vi "error_messages.vi"(8 "error in (no error)":errorcluster) -> ()   [LabVIEW 2015]
uses:
  <vilib>/Utility/error.llb/DialogType.ctl
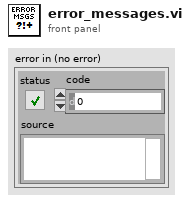
[diagram p1: front panel]
types:
  T1 = typedef "DialogType.ctl" = u16
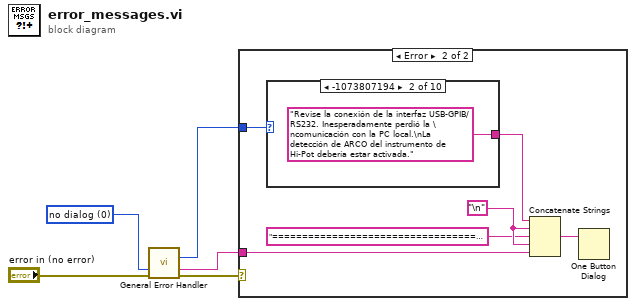
[diagram p0: block diagram]
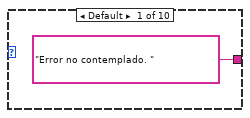
[diagram p3: hidden frame]
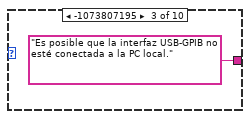
[diagram p4: hidden frame]
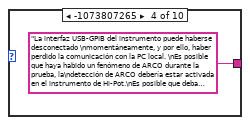
[diagram p5: hidden frame]
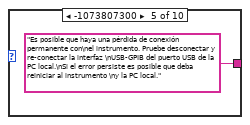
[diagram p6: hidden frame]
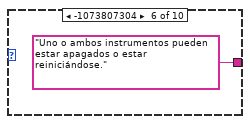
[diagram p7: hidden frame]
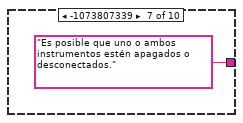
[diagram p8: hidden frame]
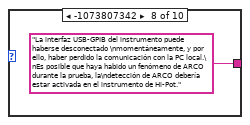
[diagram p9: hidden frame]
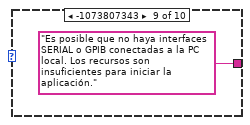
[diagram p10: hidden frame]
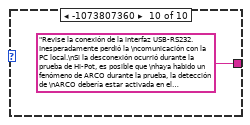
[diagram p11: hidden frame]
diagram:
  w2 = T1 0 items=["no dialog", "OK message", "continue or stop message", "OK message + warnings", "continue/stop + warnings"] ("type of dialog (OK msg:1)")
  n1 = call <vilib>:"General Error Handler.vi"("type of dialog (OK msg:1)"=w2, "error in (no error)"="error in (no error)") -> ("code out"=w4:i32, "message"=w5:string, "error out"=w3:errorcluster)  [unwired: 9 in, 2 out]
  n2 = case shown="Error" w3 {
    tunnel: w4 -> [_ w11]
    tunnel: w5 -> [_ w9]
    frame No Error {
    }
    frame Error {
      w7 = "\n"
      n3 = case shown="-1073807194" w11 {
        tunnel: ["Error no contemplado. " "Revise la conexión de la interfaz USB-GPIB/RS232. Inesperadamente perdió la \ncomunicación con la PC local.\nLa detección de ARCO del instrumento de Hi-Pot debería estar activada." "Es posible que la interfaz USB-GPIB no esté conectada a la PC local." "La interfaz USB-GPIB del instrumento puede haberse desconectado \nmomentáneamente, y por ello, haber perdido la comunicación con la PC local. \nEs posible que haya habido un fenómeno de ARCO durante la prueba, la\ndetección de ARCO debería estar activada en el instrumento de Hi-Pot.\nEs posible que deba reiniciar el instrumento y la PC local." "Es posible que haya una pérdida de conexión permanente con\nel instrumento. Pruebe desconectar y re-conectar la interfaz \nUSB-GPIB del puerto USB de la PC local.\nSi el error persiste es posible que deba reiniciar al instrumento \ny la PC local." "Uno o ambos instrumentos pueden estar apagados o estar reiniciándose." "Es posible que uno o ambos instrumentos estén apagados o desconectados." "La interfaz USB-GPIB del instrumento puede haberse desconectado \nmomentáneamente, y por ello, haber perdido la comunicación con la PC local.\nEs posible que haya habido un fenómeno de ARCO durante la prueba, la\ndetección de ARCO debería estar activada en el instrumento de Hi-Pot." "Es posible que no haya interfaces SERIAL o GPIB conectadas a la PC local. Los recursos son insuficientes para iniciar la aplicación." "Revise la conexión de la interfaz USB-RS232. Inesperadamente perdió la \ncomunicación con la PC local.\nSi la desconexión ocurrió durante la prueba de Hi-Pot, es posible que \nhaya habido un fenómeno de ARCO durante la prueba, la detección de \nARCO debería estar activada en el instrumento de Hi-Pot."] -> w10
        frame Default {
        }
        frame -1073807194 {
        }
        frame -1073807195 {
        }
        frame -1073807265 {
        }
        frame -1073807300 {
        }
        frame -1073807304 {
        }
        frame -1073807339 {
        }
        frame -1073807342 {
        }
        frame -1073807343 {
        }
        frame -1073807360 {
        }
      }
      n4 = Concatenate Strings(w10, w7, "===========================================", w7, w9) -> (w8:string)
      n5 = One Button Dialog(message=w8) -> ()  [unwired: 1 in, 1 out]
    }
  }
